vi "比例计算.vi"(0 "产品长度":dbl=23.67 format="%#_13g", 1 "产品宽度":dbl=13.3 format="%#_13g", 2 "真实X":dbl, 3 "真实Y":dbl, 6 "产品1右侧边缘X坐标":dbl, 8 "产品1左侧边缘X坐标":dbl, 10 "产品1下侧边缘Y坐标":dbl, 12 "产品1上侧边缘Y坐标":dbl) -> (14 "X":dbl format="%#.3f", 17 "Y":dbl format="%#.3f")   [LabVIEW 2020]
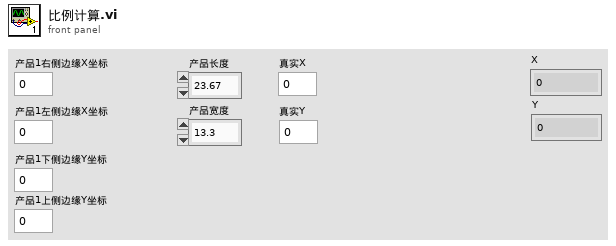
[diagram p1: front panel]
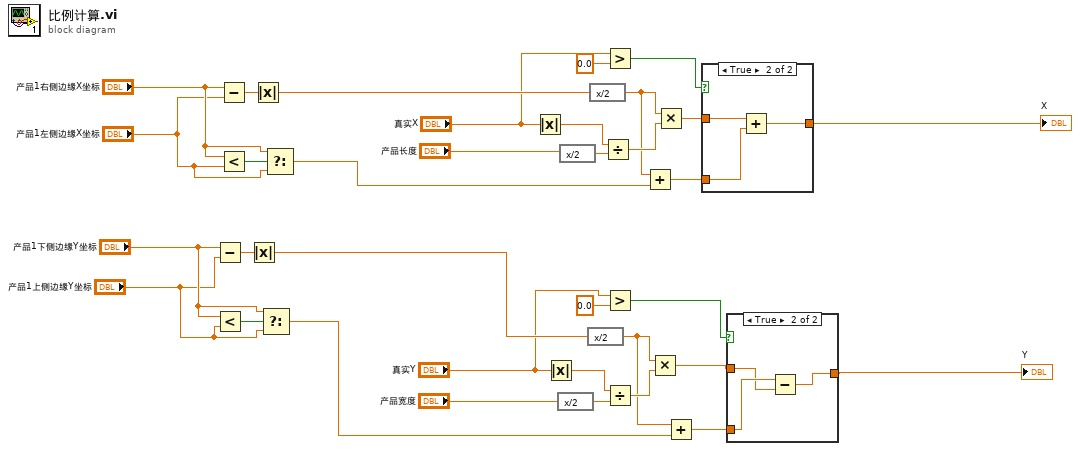
[diagram p0: block diagram]
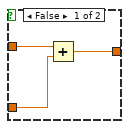
[diagram p2: hidden frame]
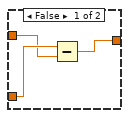
[diagram p3: hidden frame]
diagram:
  n1 = Subtract(x="产品1下侧边缘Y坐标", y="产品1上侧边缘Y坐标") -> (x-y=w20:dbl)
  n2 = Less?(x="产品1下侧边缘Y坐标", y="产品1上侧边缘Y坐标") -> (x < y?=w21:bool)
  n3 = Subtract(x="产品1右侧边缘X坐标", y="产品1左侧边缘X坐标") -> (x-y=w27:dbl)
  n4 = Less?(x="产品1右侧边缘X坐标", y="产品1左侧边缘X坐标") -> (x < y?=w25:bool)
  n5 = Absolute Value(x=w20) -> (abs(x)=w19:dbl)
  n6 = Absolute Value(x=w27) -> (abs(x)=w26:dbl)
  n7 = Select(t="产品1下侧边缘Y坐标", s=w21, f="产品1上侧边缘Y坐标") -> (s? t:f=w11:dbl)
  n8 = Select(t="产品1右侧边缘X坐标", s=w25, f="产品1左侧边缘X坐标") -> (s? t:f=w6:dbl)
  n9 = Absolute Value(x="真实X") -> (abs(x)=w13:dbl)
  n10 = Absolute Value(x="真实Y") -> (abs(x)=w1:dbl)
  n11 = expression code="x/2"("产品宽度") -> (w31:dbl)
  n12 = expression code="x/2"("产品长度") -> (w32:dbl)
  n13 = expression code="x/2"(w19) -> (w3:dbl)
  n14 = expression code="x/2"(w26) -> (w5:dbl)
  n15 = Divide(x=w13, y=w32) -> (x/y=w30:dbl)
  n16 = Greater?(x="真实X", y=0.0) -> (0:w14:bool)
  n17 = Greater?(x="真实Y", y=0.0) -> (0:w7:bool)
  n18 = Divide(x=w1, y=w31) -> (x/y=w29:dbl)
  n19 = Add(x=w5, y=w6) -> (x+y=w4:dbl)
  n20 = Multiply(x=w3, y=w29) -> (x*y=w12:dbl)
  n21 = Multiply(x=w5, y=w30) -> (x*y=w28:dbl)
  n22 = Add(x=w3, y=w11) -> (x+y=w2:dbl)
  n23 = case shown="True" w14 {
    tunnel: w28 -> [w36 w40]
    tunnel: w4 -> [w37 w39]
    tunnel: [w35 w38] -> w22
    frame False {
      n24 = Subtract(x=w37, y=w36) -> (x-y=w35:dbl)
    }
    frame True {
      n25 = Add(x=w40, y=w39) -> (x+y=w38:dbl)
    }
  }
  "X" <- w22
  n26 = case shown="True" w7 {
    tunnel: w12 -> [w43 w45]
    tunnel: w2 -> [w42 w46]
    tunnel: [w41 w44] -> w10
    frame False {
      n27 = Add(x=w43, y=w42) -> (x+y=w41:dbl)
    }
    frame True {
      n28 = Subtract(x=w46, y=w45) -> (x-y=w44:dbl)
    }
  }
  "Y" <- w10
